vi "OpenPython.vi"() -> ()   [LabVIEW 2018]
doc: "本范例演示如何调用Python函数并将双精度浮点数作为参数传递。它使用python函数来计算两个双精度浮点数之和。"
uses:
  D:/labview/LabVIEW 2018/examples/Connectivity/Python/support/PythonVersionsEnum.ctl
panel:
  out "error out":cluster{"状态":bool, "代码":i32, "源":string} caption="错误输出"
  out "a + b":dbl
  in  "b":dbl=1.0
  in  "a":dbl=41.0
  in  "error in (no error)":cluster{"状态":bool, "代码":i32, "源":string} caption="错误输入（无错误）"
  in  "Python版本":T1
  # "概述：演示调用Python函数并将双精度浮点数作为参数传递的方法。\n要求：Python 2.7或3.6，位数须与LabVIEW的位数一致。\n操作步骤：\n1.将Python版本设置为要执行代码的Python版本。\n2.运行VI。显示控件\"a + b\"中应显示\"a\"、\"b\"之和的结果。\n3.关于python节点调用如何传递参数及处理返回值的详细信息，见本VI程序框图和\"ExamplePythonModule.py\"中的注释。"
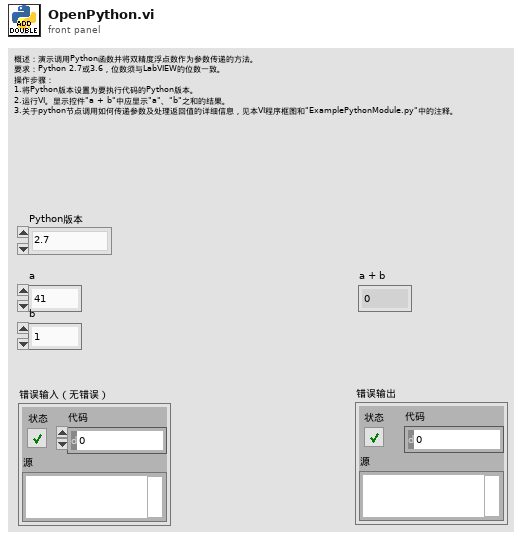
[diagram p1: front panel]
types:
  T1 = typedef "PythonVersionsEnum.ctl" = enum16{"2.7", "3.6"}
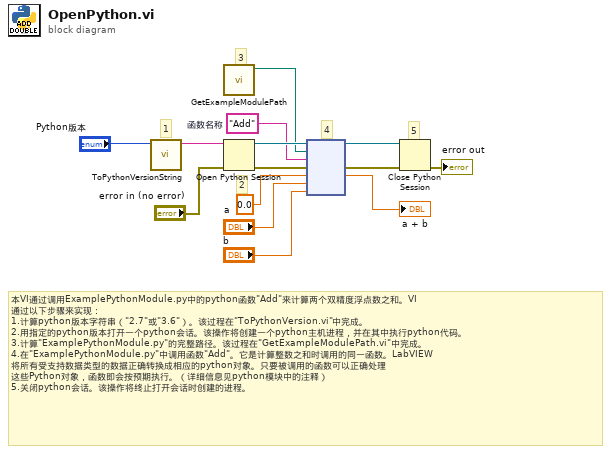
[diagram p0: block diagram]
diagram:
  w8 = "Add"  # 函数名称
  # "5"
  # "4"
  # "2"
  # "3"
  # "1"
  # "本VI通过调用ExamplePythonModule.py中的python函数\"Add\"来计算两个双精度浮点数之和。VI\n通过以下步骤来实现：\n1.计算python版本字符串（\"2.7\"或\"3.6\"）。该过程在\"ToPythonVersion.vi\"中完成。\n2.用指定的python版本打开一个python会话。该操作将创建一个python主机进程，并在其中执行python代码。\n3.计算\"ExamplePythonModule.py\"的完整路径。该过程在\"GetExampleModulePath.vi\"中完成。\n4.在\"ExamplePythonModule.py\"中调用函数\"Add\"。它是计算整数之和时调用的同一函数。LabVIEW\n将所有受支持数据类型的数据正确转换成相应的python对象。只要被调用的函数可以正确处理\n这些Python对象，函数即会按预期执行。（详细信息见python模块中的注释）\n5.关闭python会话。该操作将终止打开会话时创建的进程。"
  n1 = call "ToPythonVersionString.vi"("Python版本"="Python版本") -> ("python版本字符串"=w14:string)  [unwired: 10 in]
  n2 = call "GetExampleModulePath.vi"() -> ("模块路径"=w9:path)  [unwired: 11 in]
  n3 = Open Python Session(python version=w14, 3:"error in (no error)") -> (session out=w11:refnum<k35>, error out=w10:errorcluster)  [unwired: 1 in]
  n4 = node(w11, w9, w8, w10, 0.0 ("a"), "a", "b") -> (w7:refnum<k35>, w6:errorcluster, →"a + b":dbl)  [unwired: 2 in, 2 out]
  n5 = Close Python Session(session in=w7, error in=w6) -> (11:→"error out":errorcluster)
